vi "CRCL.vi"() -> ()   [LabVIEW 2013]
uses:
  ROS/Code/SubVIs/BaxterSide.ctl
  NIST2/Arm Globals.vi
  ROS/Code/Console/Servers/ServerSubs/(nist) Arm Globals.vi
  NIST2/Prim/Fwd Kenimatics - array.vi
  <vilib>/Analysis/Matrix/Numeric/Multiply/Multiply - RM,R.vi
  <vilib>/Analysis/Matrix/NI_Matrix.lvlib
panel:
  out "pose":dbl[][](array[numeric])
  out "R:Joints":dbl[](array[numeric])=[-0.416, -0.52, 1.12, -3.856, -0.084, -0.176, 0.14]
  in  "Status":T1={"Canon"=FALSE, "Speed"=0.0, "Axis Speed"=0.0, "Use Degrees"=FALSE, "Relative Speed"=0.0, "Length Unit Adj"=1.0} {"Length Unit Adj" format="%.2f"; "Relative Speed" format="%.2f"}
  out "Response":i32=3
  in  "Command":string
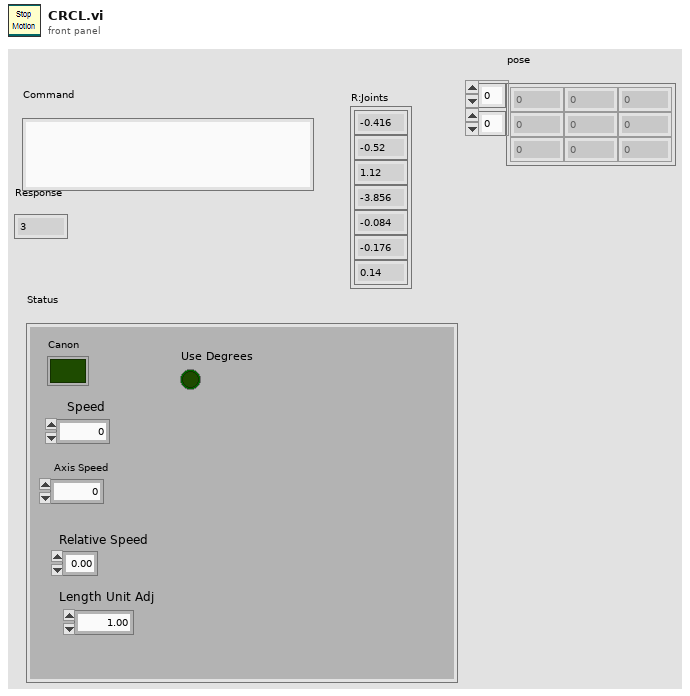
[diagram p1: front panel]
types:
  T1 = cluster{"Canon":bool, "Speed":dbl, "Axis Speed":dbl, "Use Degrees":bool, "Relative Speed":dbl, "Length Unit Adj":dbl}
  T2 = typedef "BaxterSide.ctl" = enum16{"left", "right"}
  T3 = typedef "NI_Matrix.lvlib/RealMatrix.ctl" = dbl[][]
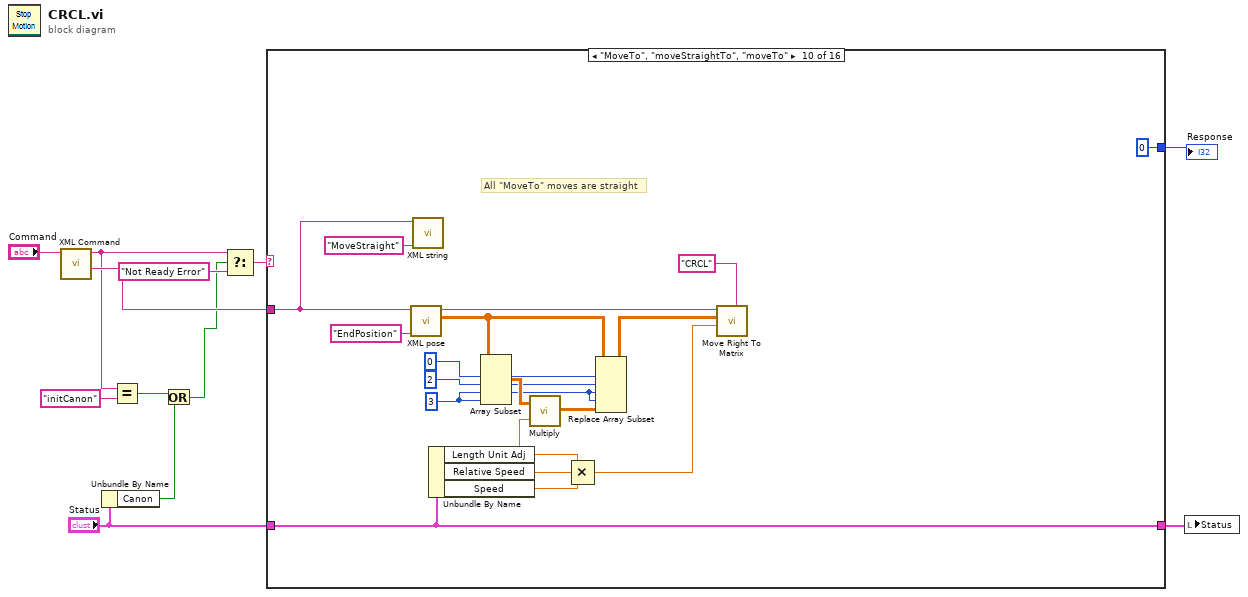
[diagram p0: block diagram]
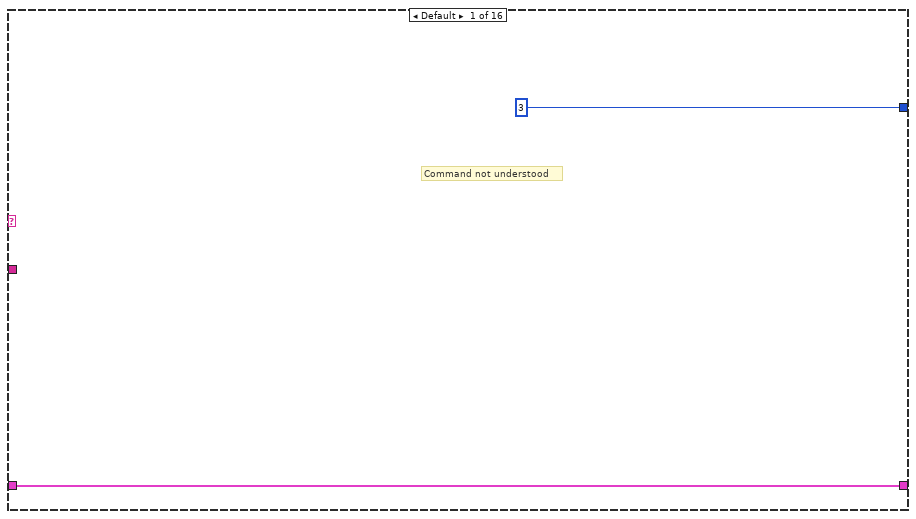
[diagram p2: hidden frame]
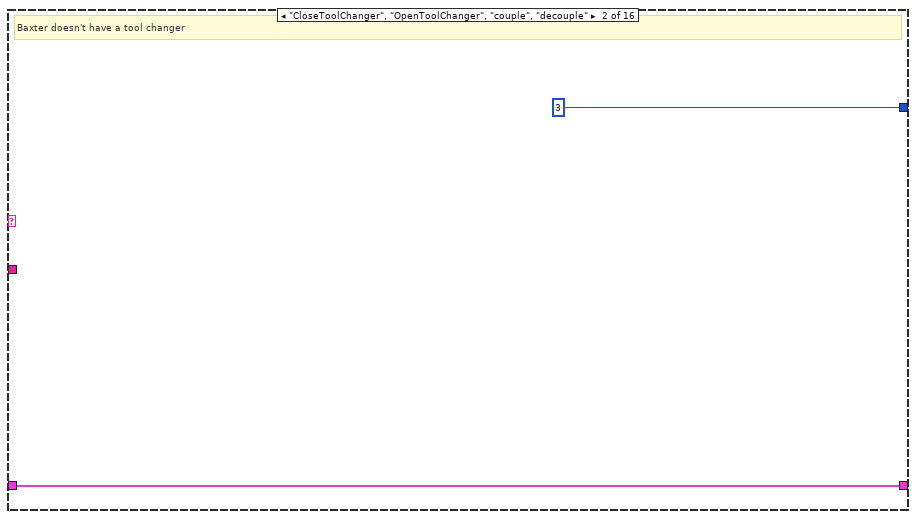
[diagram p3: hidden frame]
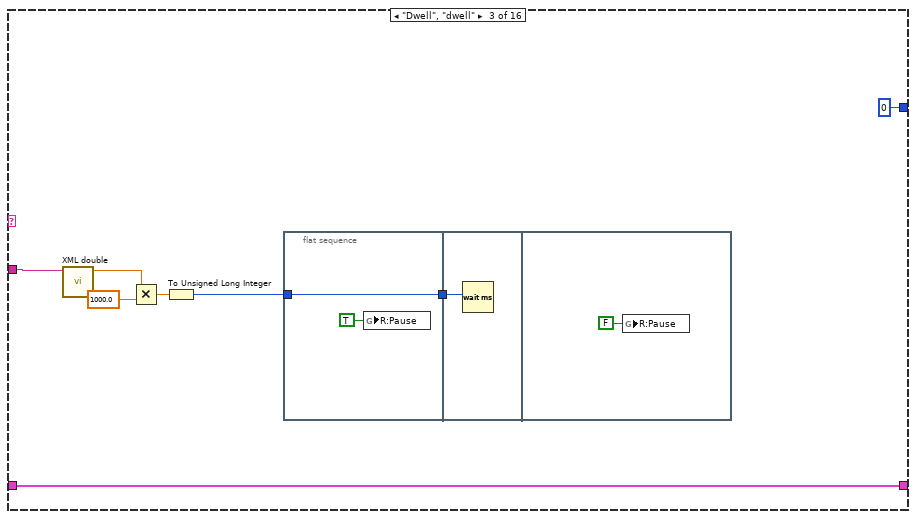
[diagram p4: hidden frame]
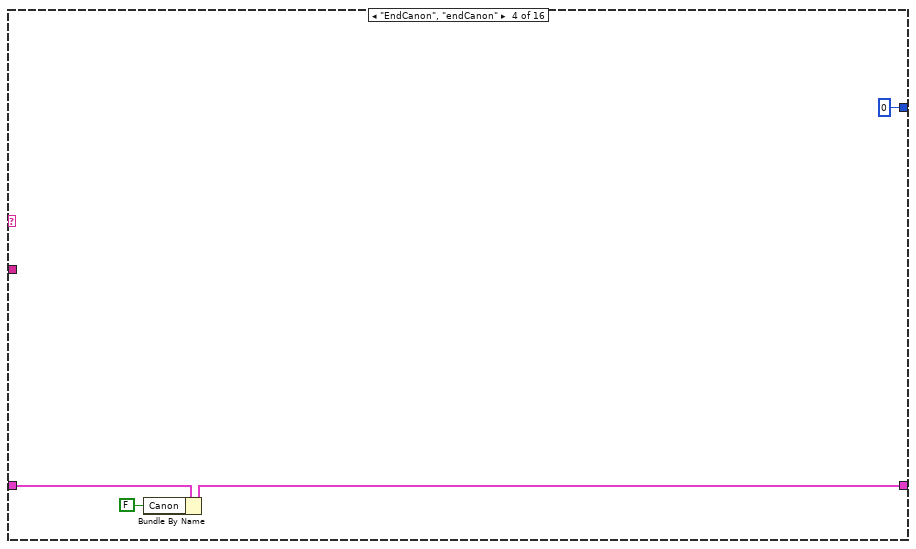
[diagram p5: hidden frame]
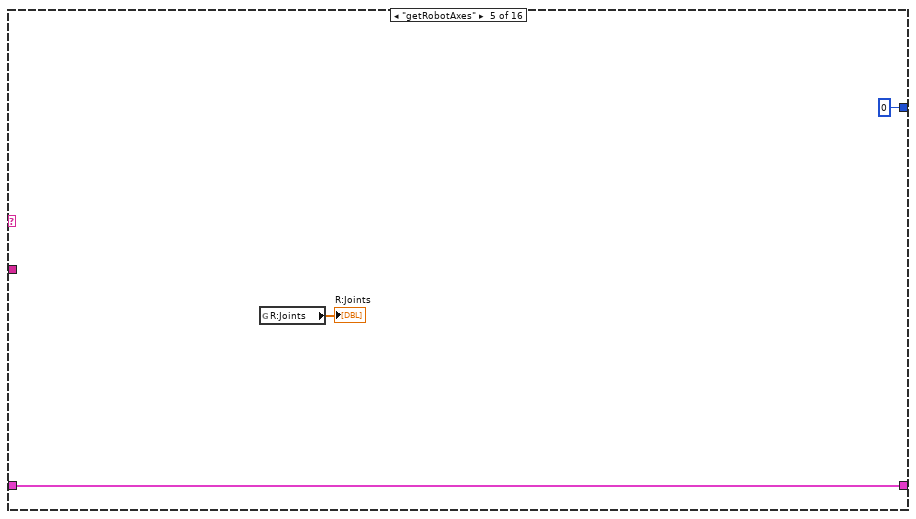
[diagram p6: hidden frame]
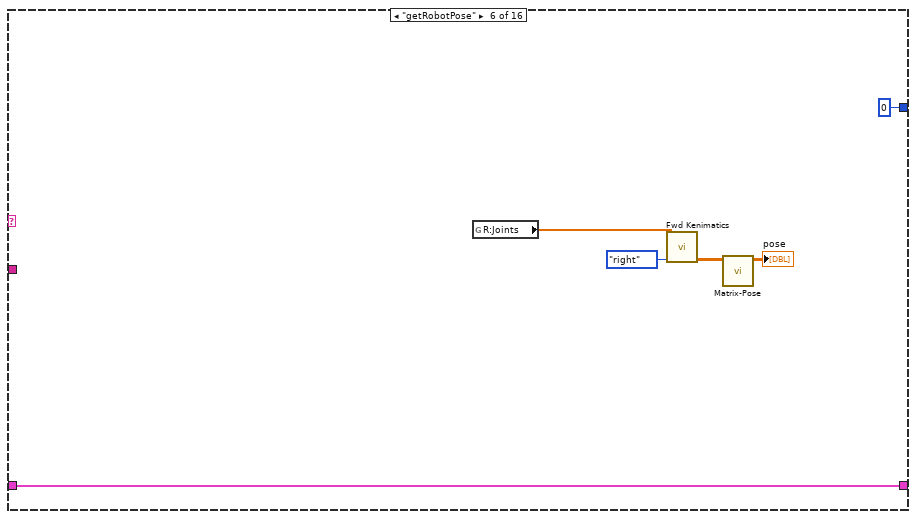
[diagram p7: hidden frame]
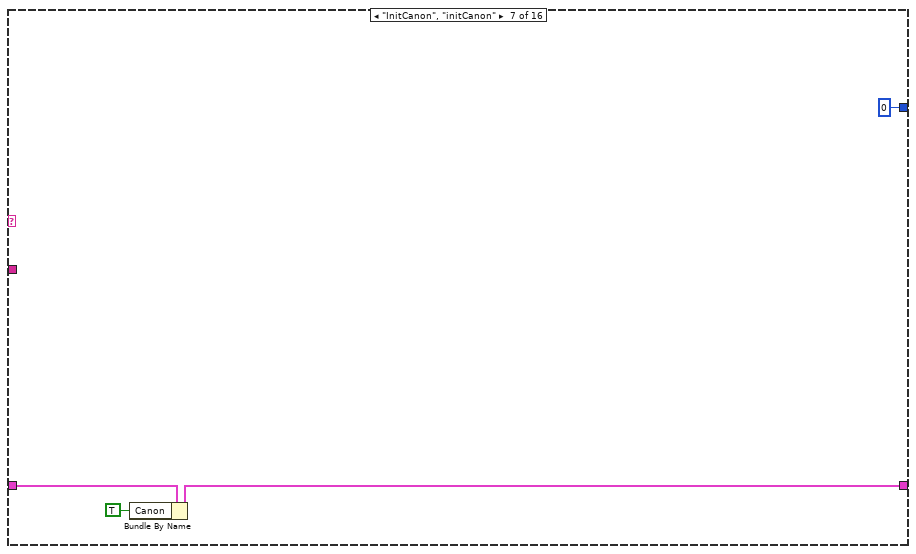
[diagram p8: hidden frame]
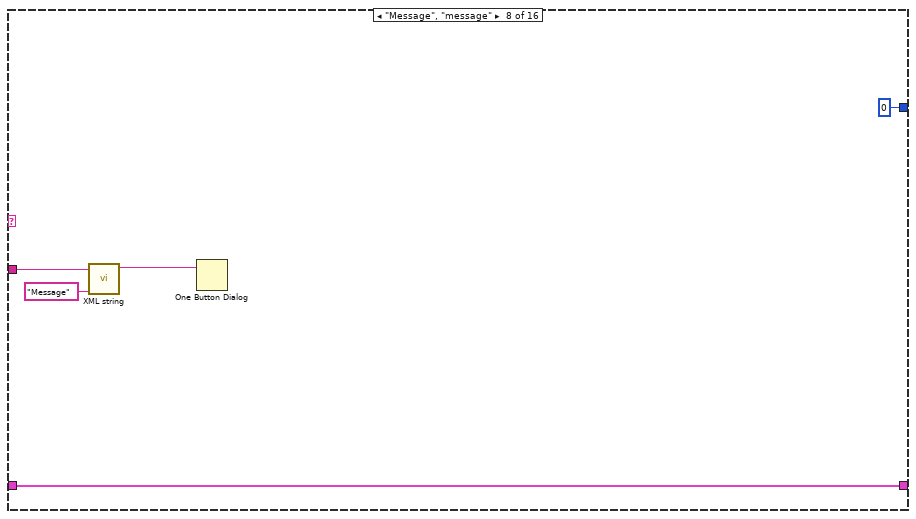
[diagram p9: hidden frame]
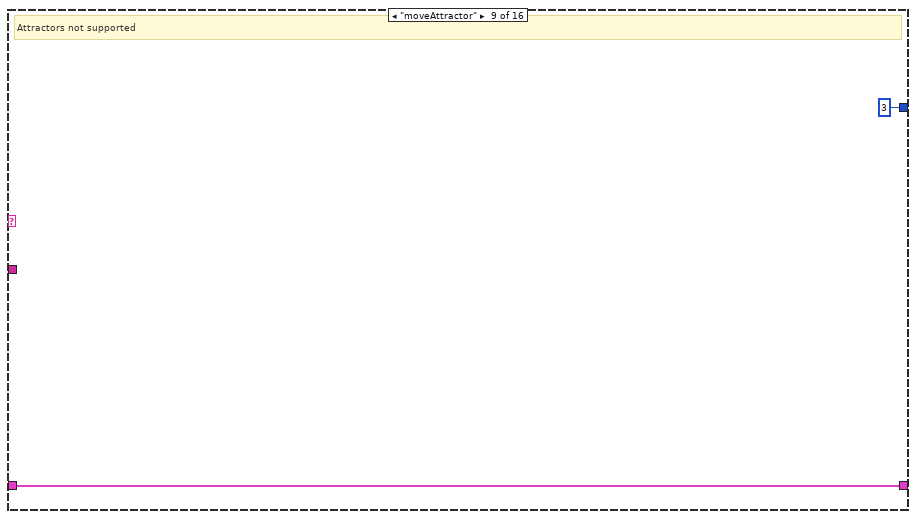
[diagram p10: hidden frame]
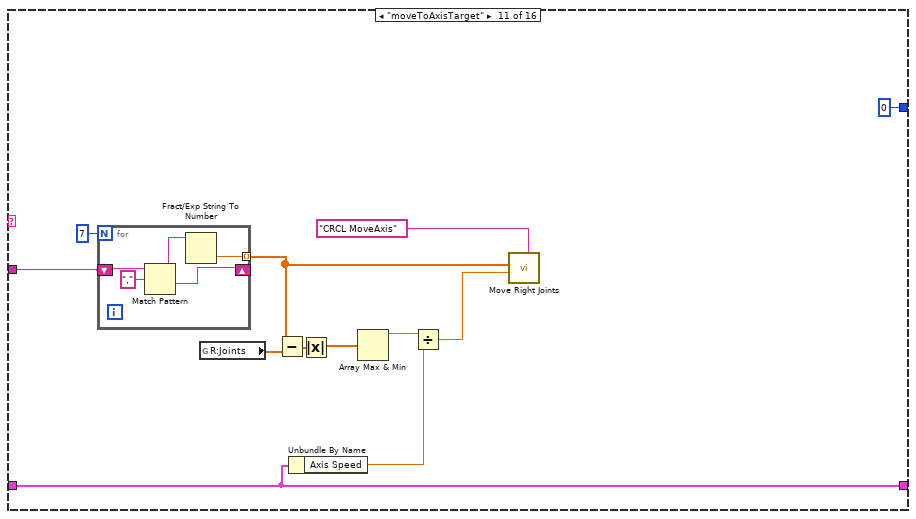
[diagram p11: hidden frame]
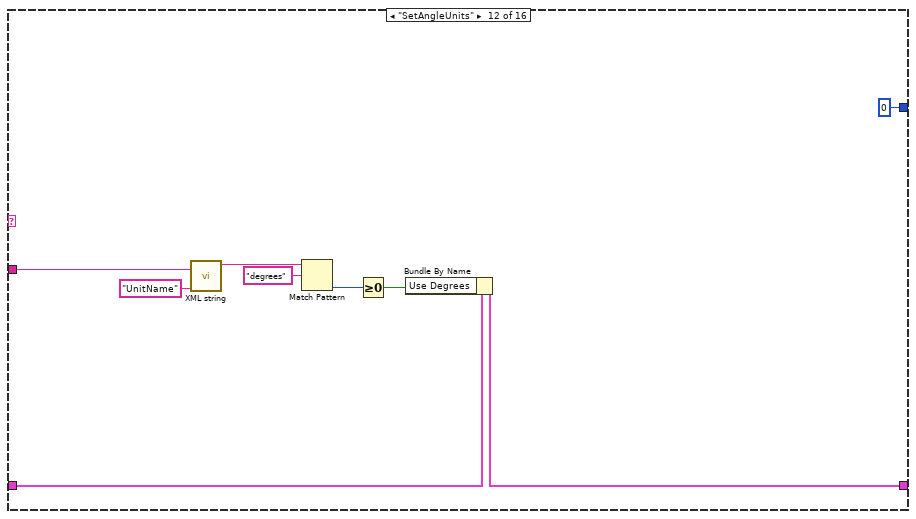
[diagram p12: hidden frame]
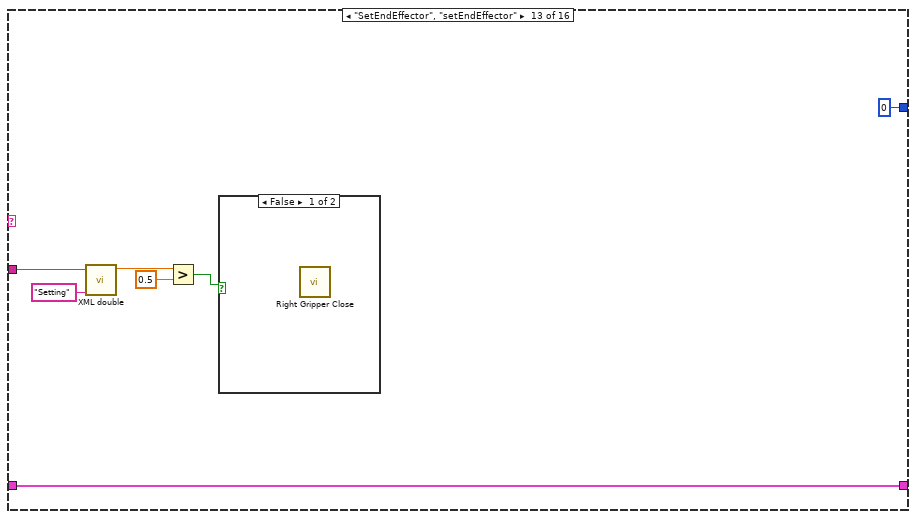
[diagram p13: hidden frame]
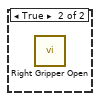
[diagram p14: hidden frame]
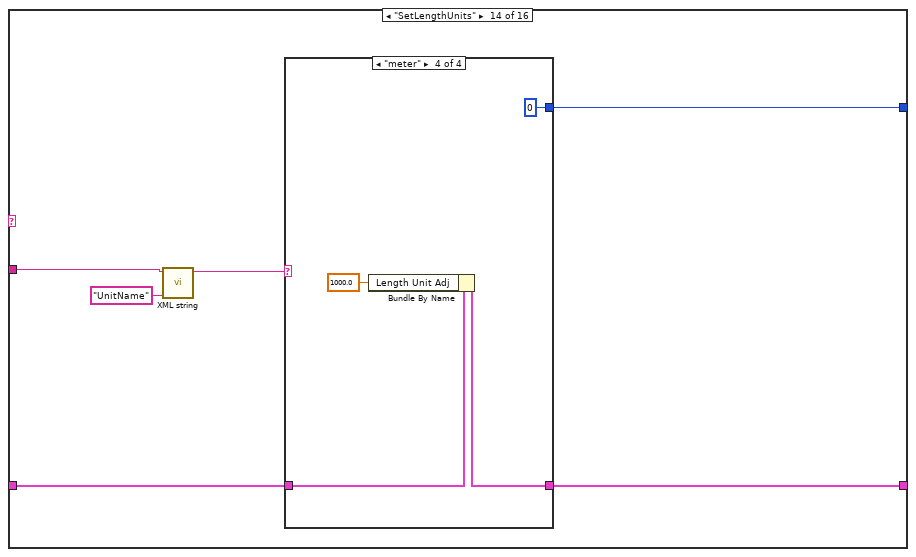
[diagram p15: hidden frame]
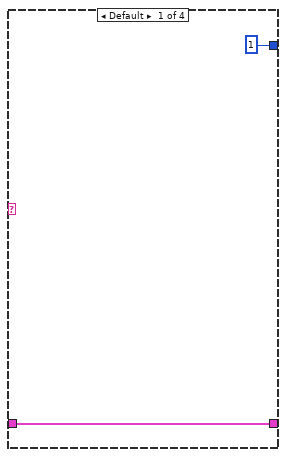
[diagram p16: hidden frame]
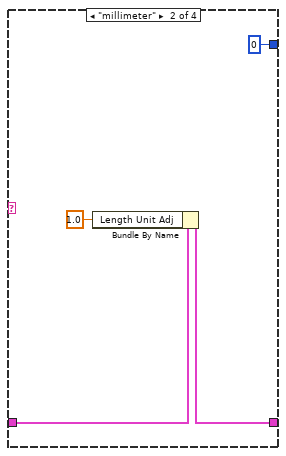
[diagram p17: hidden frame]
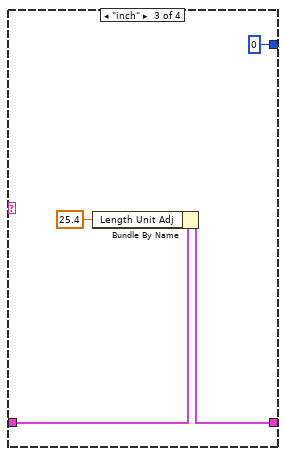
[diagram p18: hidden frame]
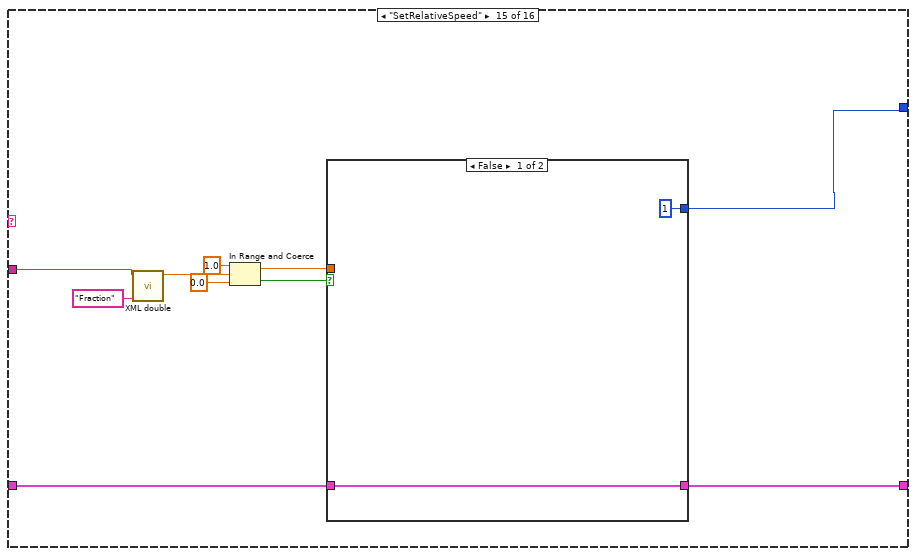
[diagram p19: hidden frame]
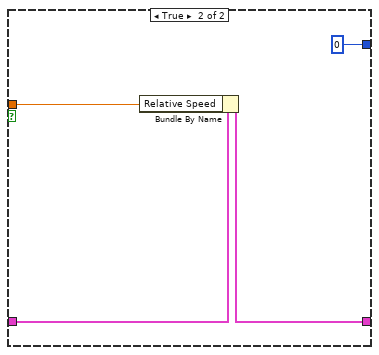
[diagram p20: hidden frame]
diagram:
  n1 = call "XML Command.vi"("String"="Command") -> ("Parameters"=w3:string, "Command"=w2:string)  [unwired: 8 in, 1 out]
  n2 = Unbundle By Name("Status") -> ("Canon"=w5:bool)
  n3 = Equal?(x=w2, y="initCanon") -> (x = y?=w6:bool)
  n4 = Or(x=w6, y=w5) -> (x .or. y?=w1:bool)
  n5 = Select(t=w2, s=w1, f="Not Ready Error") -> (s? t:f=w11:string)
  n6 = case shown="\"MoveTo\", \"moveStraightTo\", \"moveTo\"" w11 {
    tunnel: [3 3 0 0 0 0 0 0 3 0 0 0 0 w106 w124 0] -> w10
    tunnel: w3 -> [_ _ w22 _ _ _ _ w48 _ w66 w79 w94 w101 w108 w133 w145]
    tunnel: "Status" -> [w13 w15 w23 w32 w33 w41 w45 w50 w51 w69 w76 w95 w102 w105 w126 w143]
    tunnel: [w13 w15 w23 w30 w33 w41 w43 w50 w51 w69 w76 w92 w102 w104 w125 w142] -> w8
    frame Default {
      # "Command not understood"
    }
    frame "CloseToolChanger", "OpenToolChanger", "couple", "decouple" {
      # "Baxter doesn't have a tool changer"
    }
    frame "Dwell", "dwell" {
      n7 = call "XML double.vi"("String"=w22) -> ("int"=w21:dbl)  [unwired: 10 in]
      n8 = Multiply(x=w21, y=1000.0) -> (x*y=w19:dbl)
      n9 = To Unsigned Long Integer(number=w19) -> (unsigned 32bit integer=w17:u32)
      n10 = flat-sequence {
        tunnel: [w25] -> w18
        tunnel: w17 -> [w25]
        tunnel: w18 -> [w27]
        frame #0 {
          n11 = global write "Arm Globals.vi" "R:Pause"(TRUE ("R:Pause")) -> ()
        }
        frame #1 {
          n12 = Wait (ms)(milliseconds to wait=w27) -> ()  [unwired: 1 out]
        }
        frame #2 {
          n13 = global write "Arm Globals.vi" "R:Pause"(FALSE ("R:Pause")) -> ()
        }
      }
    }
    frame "EndCanon", "endCanon" {
      n14 = Bundle By Name(cluster=w32, "Canon"=FALSE) -> (w30:T1)
    }
    frame "getRobotAxes" {
      n15 = global read "(nist) Arm Globals.vi" "R:Joints"() -> (→"R:Joints":dbl[])
    }
    frame "getRobotPose" {
      n16 = global read "(nist) Arm Globals.vi" "R:Joints"() -> (w38:dbl[])
      n17 = call-poly "Fwd Kenimatics.vi"("Side"=BaxterSide."right", "Joints"=w38) -> ("Matrix"=w39:T3)  [unwired: 8 in, 1 out]
      n18 = call "Matrix-Pose.vi"("T"=w39) -> ("pose"=→"pose":dbl[][])  [unwired: 9 in, 1 out]
    }
    frame "InitCanon", "initCanon" {
      n19 = Bundle By Name(cluster=w45, "Canon"=TRUE) -> (w43:T1)
    }
    frame "Message", "message" {
      n20 = call "XML string.vi"("tag"="Message", "String"=w48) -> ("string"=w46:string)  [unwired: 8 in, 1 out]
      n21 = One Button Dialog(message=w46) -> ()  [unwired: 1 in, 1 out]
    }
    frame "moveAttractor" {
      # "Attractors not supported"
    }
    frame "MoveTo", "moveStraightTo", "moveTo" {
      w56 = 3 ("column 1")
      w57 = 2 ("row N")
      w58 = 0 ("row 1")
      # "All \"MoveTo\" moves are straight"
      n22 = call "XML pose.vi"("tag"="EndPosition", "String"=w66) -> ("T"=w54:T3, "Object"=w67:string)  [unwired: 7 in, 1 out]
      n23 = call "XML string.vi"("tag"="MoveStraight", "String"=w66) -> ()  [unwired: 8 in, 2 out]
      n24 = Unbundle By Name(w69) -> ("Length Unit Adj"=w59:dbl, "Relative Speed"=w63:dbl, "Speed"=w62:dbl)
      n25 = Array Subset(array=w54, index (row)=w58, length (row)=w57, index (col)=w56, length (col)=w56) -> (w60:T3)
      n26 = call-poly <vilib>:"Multiply.vi"("Real Scalar c"=w59, "Real Matrix A"=w60) -> ("A * c"=w55:T3)
      n27 = Compound Arithmetic op=MULTIPLY(w59, w63, w62) -> (w61:dbl)
      n28 = Replace Array Subset(array=w54, new element=w55, index (dim 0)=w58, index (dim 1)=w57, index (dim 2)=w56, index (dim 3)=w56) -> (w53:T3)
      n29 = call "Move Right To Matrix.vi"("Label"="CRCL", "Speed (mm/s)"=w61, "Goal Pose in Location"=w53, "Location"=w67) -> ()  [unwired: 7 in, 1 out]
    }
    frame "moveToAxisTarget" {
      n30 = for {
        N: 7 -> [_]
        shift-right: [w84] -> _
        shift-left: w79 -> [w87]
        tunnel: [w83] -> w78 mode=indexing
        n31 = Match Pattern(string=w87, regular expression=",") -> (before substring=w85:string, after substring=w84:string)  [unwired: 1 in, 2 out]
        n32 = Fract/Exp String To Number(string=w85) -> (number=w83:dbl)  [unwired: 3 in, 1 out]
      }
      n33 = global read "(nist) Arm Globals.vi" "R:Joints"() -> (w71:dbl[])
      n34 = Subtract(x=w78, y=w71) -> (x-y=w72:dbl[])
      n35 = Unbundle By Name(w76) -> ("Axis Speed"=w74:dbl)
      n36 = Absolute Value(x=w72) -> (abs(x)=w77:dbl[])
      n37 = Array Max & Min(array=w77) -> (max value=w75:dbl)  [unwired: 3 out]
      n38 = Divide(x=w75, y=w74) -> (x/y=w73:dbl)
      n39 = call "Move Right Joints.vi"("Label"="CRCL MoveAxis", "time"=w73, "Goal"=w78) -> ()  [unwired: 8 in, 1 out]
    }
    frame "SetAngleUnits" {
      n40 = call "XML string.vi"("tag"="UnitName", "String"=w94) -> ("string"=w91:string)  [unwired: 8 in, 1 out]
      n41 = Match Pattern(string=w91, regular expression="degrees") -> (offset past match=w89:i32)  [unwired: 1 in, 3 out]
      n42 = Greater Or Equal To 0?(x=w89) -> (x >= 0?=w88:bool)
      n43 = Bundle By Name(cluster=w95, "Use Degrees"=w88) -> (w92:T1)
    }
    frame "SetEndEffector", "setEndEffector" {
      n44 = call "XML double.vi"("tag"="Setting", "String"=w101) -> ("int"=w99:dbl)  [unwired: 9 in]
      n45 = Greater?(x=w99, y=0.5) -> (0:w97:bool)
      n46 = case shown="False" w97 {
        frame False {
          n47 = call "Right Gripper Close.vi"() -> ()  [unwired: 10 in, 2 out]
        }
        frame True {
          n48 = call "Right Gripper Open.vi"() -> ()  [unwired: 11 in, 1 out]
        }
      }
    }
    frame "SetLengthUnits" {
      n49 = call "XML string.vi"("tag"="UnitName", "String"=w108) -> ("string"=w107:string)  [unwired: 8 in, 1 out]
      n50 = case shown="\"meter\"" w107 {
        tunnel: [1 0 0 0] -> w106
        tunnel: w105 -> [w110 w114 w118 w122]
        tunnel: [w110 w113 w117 w121] -> w104
        frame Default {
        }
        frame "millimeter" {
          n51 = Bundle By Name(cluster=w114, "Length Unit Adj"=1.0) -> (w113:T1)
        }
        frame "inch" {
          n52 = Bundle By Name(cluster=w118, "Length Unit Adj"=25.4) -> (w117:T1)
        }
        frame "meter" {
          n53 = Bundle By Name(cluster=w122, "Length Unit Adj"=1000.0) -> (w121:T1)
        }
      }
    }
    frame "SetRelativeSpeed" {
      n54 = call "XML double.vi"("tag"="Fraction", "String"=w133) -> ("int"=w131:dbl)  [unwired: 9 in]
      n55 = In Range and Coerce(upper limit=1.0, x=w131, lower limit=0.0) -> (coerced(x)=w127:dbl, In Range?=w128:bool)
      n56 = case shown="False" w128 {
        tunnel: w127 -> [_ w137]
        tunnel: w126 -> [w134 w139]
        tunnel: [w134 w138] -> w125
        tunnel: [1 0] -> w124
        frame False {
        }
        frame True {
          n57 = Bundle By Name(cluster=w139, "Relative Speed"=w137) -> (w138:T1)
        }
      }
    }
    frame "SetAbsoluteSpeed" {
      n58 = call "XML double.vi"("tag"="Speed", "String"=w145) -> ("int"=w140:dbl)  [unwired: 9 in]
      n59 = Bundle By Name(cluster=w143, "Speed"=w140) -> (w142:T1)
    }
  }
  "Response" <- w10
  n60 = local write "Status"(w8) -> ()
